vi "_Set All DAC Values.vi"(3 "Control CH":u8, 4 "Record Values (F)":bool, 5 "Load DAC(T)":bool=TRUE, 6 "DAC Value Offset (70)":u16=70, 7 "Channel ID Offset (10)":u16=10, 8 "# of Active Channels":u16) -> (0 "DACS":u32)   [LabVIEW 2015]
uses:
  <vilib>/rvi/Memory/Memory_Emulation/nirvimemoryEmulation.vi
  <vilib>/rvi/Memory/Memory_Emulation/nirvimemoryFastEmulation.vi
  <vilib>/rvi/DataTransferAndStorage/Container/Common/niFpgaContainerGetUniqueNameForEmu.vi
  <vilib>/rvi/Memory/Memory_Emulation/niFpgaMemoryEmulationCacheClearOnFirstRun.vi
  <vilib>/rvi/Memory/Memory_Emulation/nirvimemoryEmulationManagerCache_MakeExclusive.vi
  <vilib>/rvi/Memory/Memory_Emulation/niFpgaMemoryEmulationValidateCache.vi
  <vilib>/rvi/Memory/Memory_Emulation/nirvimemoryEmulationManagerCache_InsertValue.vi
  <vilib>/Utility/error.llb/Clear Errors.vi
  <vilib>/rvi/Memory/Memory_Emulation/nirvimemoryEmulationManagerCache_ReleaseExclusive.vi
  <vilib>/rvi/Memory/Memory_Emulation/nirvimemoryEmulationManagerCache_GetValue.vi
  <vilib>/rvi/Emulation/niFpgaEmulationIsFPGAContextNoSignature.vi
  <vilib>/rvi/Emulation/niFpgaSctlEmulationGetInTimedLoop.vi
  <vilib>/rvi/Memory/Memory_Emulation/nirvimemoryEmulationManagerCache_SetValue.vi
  <vilib>/rvi/Emulation/niFpgaSctlEmulationResourceMgr.vi
  <vilib>/rvi/DataTransferAndStorage/Container/XNode/niFpgaContainer.xnode
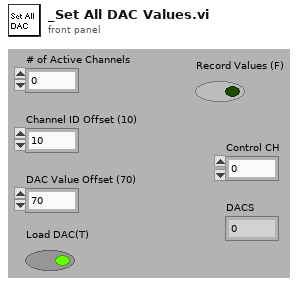
[diagram p1: front panel]
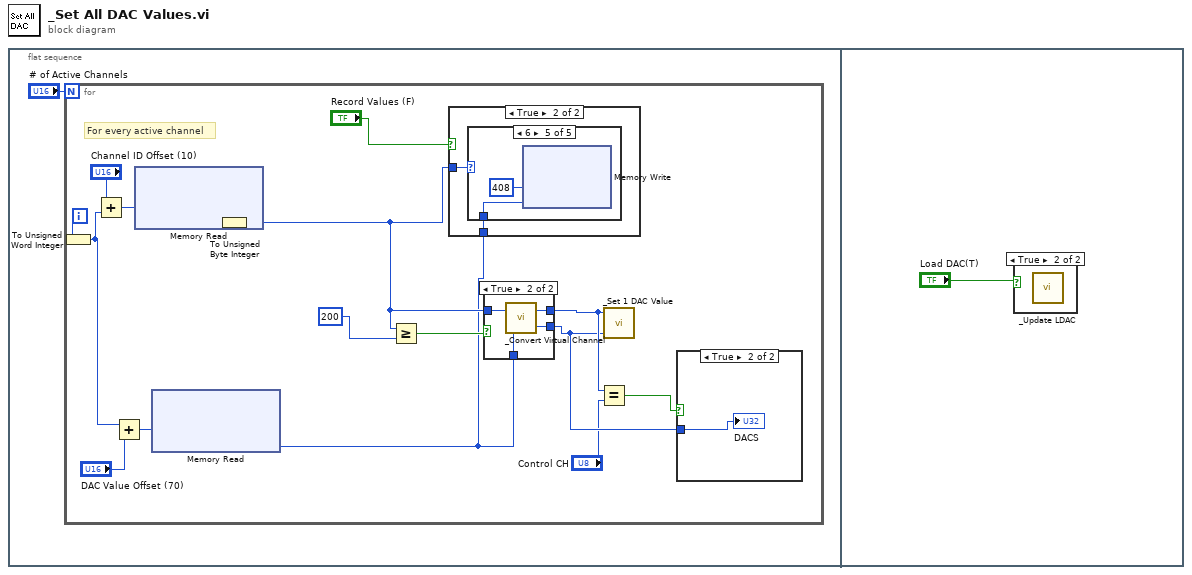
[diagram p0: block diagram]
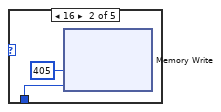
[diagram p5: hidden frame]
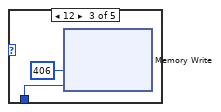
[diagram p6: hidden frame]
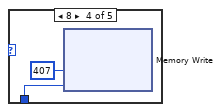
[diagram p7: hidden frame]
diagram:
  n1 = flat-sequence {
    frame #0 {
      n2 = for {
        N: "# of Active Channels" -> [_]
        i -> [w17]
        # "For every active channel"
        n3 = To Unsigned Word Integer(number=w17) -> (unsigned 16bit integer=w13:u16)
        n4 = Add(x="Channel ID Offset (10)", y=w13) -> (x+y=w11:u16)
        n5 = Add(x=w13, y="DAC Value Offset (70)") -> (x+y=w14:u16)
        n6 = xnode ("Memory Read")("Address"=w11) -> ("Data"=w12:u32)  [unwired: 1 in, 1 out]
        n7 = xnode ("Memory Read")("Address"=w14) -> ("Data"=w6:u32)  [unwired: 1 in, 1 out]
        n8 = To Unsigned Byte Integer(number=w12) -> (unsigned 8bit integer=w7:u8)
        n9 = Greater Or Equal?(x=w7, y=u8 200) -> (x >= y?=w9:bool)
        n10 = case shown="True" "Record Values (F)" {
          tunnel: w7 -> [_ w20]
          tunnel: w6 -> [_ w19]
          frame False {
          }
          frame True {
            n11 = case shown="6" w20 {
              tunnel: w19 -> [_ w21 w23 w25 w27]
              frame 0, Default {
              }
              frame 16 {
                n12 = xnode ("Memory Write")("Address"=u32 405, "Data"=w21) -> ()  [unwired: 1 in, 1 out]
              }
              frame 12 {
                n13 = xnode ("Memory Write")("Address"=u32 406, "Data"=w23) -> ()  [unwired: 1 in, 1 out]
              }
              frame 8 {
                n14 = xnode ("Memory Write")("Address"=u32 407, "Data"=w25) -> ()  [unwired: 1 in, 1 out]
              }
              frame 6 {
                n15 = xnode ("Memory Write")("Address"=u32 408, "Data"=w27) -> ()  [unwired: 1 in, 1 out]
              }
            }
          }
        }
        n16 = case shown="True" w9 {
          tunnel: [w30 w34] -> w5
          tunnel: w6 -> [w29 w33]
          tunnel: [w29 w32] -> w3
          tunnel: w7 -> [w30 w31]
          frame False {
          }
          frame True {
            n17 = call "_Convert Virtual Channel.vi"("DAC"=w33, "Ch#"=w31) -> ("DAC Out"=w32:u32, "Ch# Out"=w34:u8)
          }
        }
        n18 = Equal?(x=w5, y="Control CH") -> (x = y?=w4:bool)
        n19 = call "_Set 1 DAC Value.vi"("DAC"=w3, "Ch#"=w5) -> ()  [unwired: 2 out]
        n20 = case shown="True" w4 {
          tunnel: w3 -> [_ w18]
          frame False {
          }
          frame True {
            "DACS" <- w18
          }
        }
      }
    }
    frame #1 {
      n21 = case shown="True" "Load DAC(T)" {
        frame False {
        }
        frame True {
          n22 = call "_Update LDAC.vi"() -> ()  [unwired: 6 out]
        }
      }
    }
  }
